vi "Test - Add  Property (Array).vi"() -> ()   [LabVIEW 2020, in "JSON Schema Generator.lvlib"]
uses:
  JSON Schema Generator.lvlib
  <vilib>/addons/_JKI Toolkits/Caraya/classes/Test/Test.lvclass
  <vilib>/addons/_JKI Toolkits/Caraya/classes/Assert/Assert.lvclass
  <vilib>/addons/_JKI Toolkits/Caraya/classes/Assert/Assert Not Error.vi
  <vilib>/JDP Science/JSONtext/JSONtext.lvlib
  <vilib>/addons/_JKI Toolkits/Caraya/classes/Assert/Assert Equal Value_Variant.vi
panel:
  in  "Array 2":string[](array[string])
  in  "Array":T1(array[cluster])
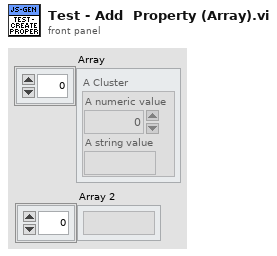
[diagram p1: front panel]
types:
  T1 = cluster{"A numeric value":i32, "A string value":string}[]
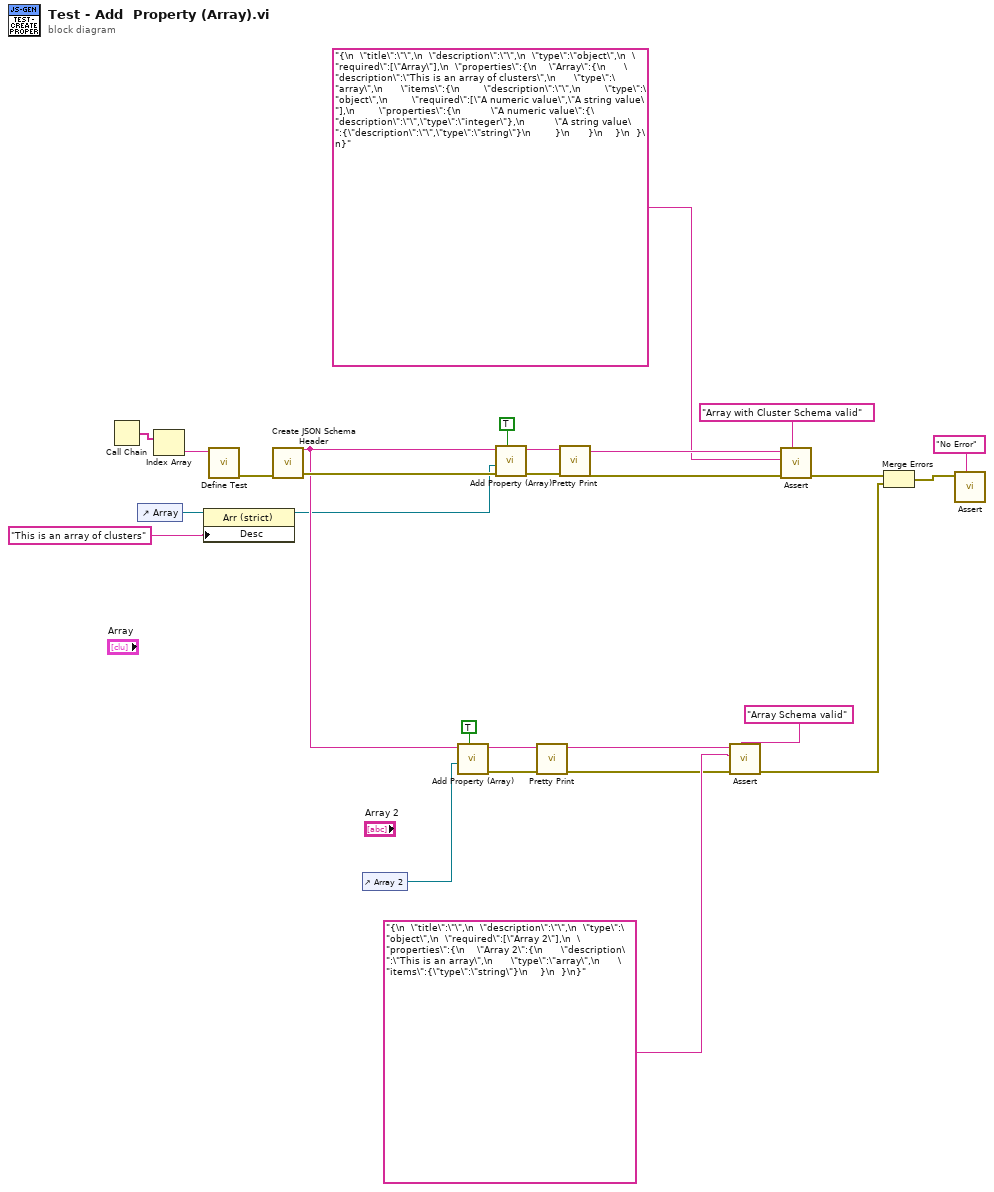
[diagram p0: block diagram]
diagram:
  n1 = Call Chain() -> (call chain=w27:string[])
  n2 = control-ref of="Array"() -> (w7:refnum<vi>)
  n3 = Index Array(array=w27) -> (element=w26:string)  [unwired: 1 in]
  n4 = property class="Arr (strict)"(reference=w7, "Desc"="This is an array of clusters" ("Description")) -> (reference out=w2:refnum<vi>)  [unwired: 1 in, 1 out]
  n5 = call <vilib>:"Define Test.vi"("Label (VI Title)"=w26) -> ("error out"=w21:errorcluster)  [unwired: 9 in, 1 out]
  n6 = call "Create JSON Schema Header.vi"("error in (no error)"=w21) -> ("error out"=w16:errorcluster, "JSON Schema out"=w12:string)  [unwired: 9 in]
  n7 = control-ref of="Array 2"() -> (w6:refnum<vi>)
  n8 = call "Add Property (Array).vi"("Required?"=TRUE, "Array Ref in"=w6, "JSON Schema in"=w12) -> ("error out"=w9:errorcluster, "JSON SChema out"=w4:string)  [unwired: 7 in]
  n9 = call "Add Property (Array).vi"("Required?"=TRUE, "error in (no error)"=w16, "Array Ref in"=w2, "JSON Schema in"=w12) -> ("error out"=w18:errorcluster, "JSON SChema out"=w19:string)  [unwired: 6 in]
  n10 = call <vilib>:"Pretty Print.vi"("error in (no error)"=w9, "JSON"=w4) -> ("error out"=w5:errorcluster, "<JSON>"=w3:string)  [unwired: 7 in, 1 out]
  n11 = call <vilib>:"Pretty Print.vi"("error in (no error)"=w18, "JSON"=w19) -> ("error out"=w17:errorcluster, "<JSON>"=w15:string)  [unwired: 7 in, 1 out]
  n12 = call-poly <vilib>:"Assert.vi"("Label"="Array Schema valid", "error in (no error)"=w5, "Actual"="{\n  \"title\":\"\",\n  \"description\":\"\",\n  \"type\":\"object\",\n  \"required\":[\"Array 2\"],\n  \"properties\":{\n    \"Array 2\":{\n      \"description\":\"This is an array\",\n      \"type\":\"array\",\n      \"items\":{\"type\":\"string\"}\n    }\n  }\n}", "Expected"=w3) -> ("error out"=w8:errorcluster)  [unwired: 6 in, 1 out]
  n13 = call-poly <vilib>:"Assert.vi"("Label"="Array with Cluster Schema valid", "error in (no error)"=w17, "Actual"="{\n  \"title\":\"\",\n  \"description\":\"\",\n  \"type\":\"object\",\n  \"required\":[\"Array\"],\n  \"properties\":{\n    \"Array\":{\n      \"description\":\"This is an array of clusters\",\n      \"type\":\"array\",\n      \"items\":{\n        \"description\":\"\",\n        \"type\":\"object\",\n        \"required\":[\"A numeric value\",\"A string value\"],\n        \"properties\":{\n          \"A numeric value\":{\"description\":\"\",\"type\":\"integer\"},\n          \"A string value\":{\"description\":\"\",\"type\":\"string\"}\n        }\n      }\n    }\n  }\n}", "Expected"=w15) -> ("error out"=w24:errorcluster)  [unwired: 6 in, 1 out]
  n14 = Merge Errors(w24, w8) -> (w22:errorcluster)
  n15 = call-poly <vilib>:"Assert.vi"("Label"="No Error", "Not Error?"=w22) -> ()  [unwired: 8 in, 2 out]
